vi "Write Nested Viewable Enqueuers.vi"(8 "error in (no error)":errorcluster, 9 "Viewable Names (optional)":string[](array[string]), 10 "Nested Viewable Enqueuers":refnum<class "Message Enqueuer.lvclass">[](array[class]), 11 "IViewManager In":refnum<class "IViewManager.lvclass">) -> (0 "error out":errorcluster, 3 "IViewManager Out":refnum<class "IViewManager.lvclass">)   [LabVIEW 2018, in "MVA Framework.lvlib" / "IViewManager.lvlib" / "IViewManager.lvclass"]
doc: "写入嵌套视图消息队列"
uses:
  IViewManager.lvclass
  <vilib>/ActorFramework/Message Enqueuer/Message Enqueuer.lvclass
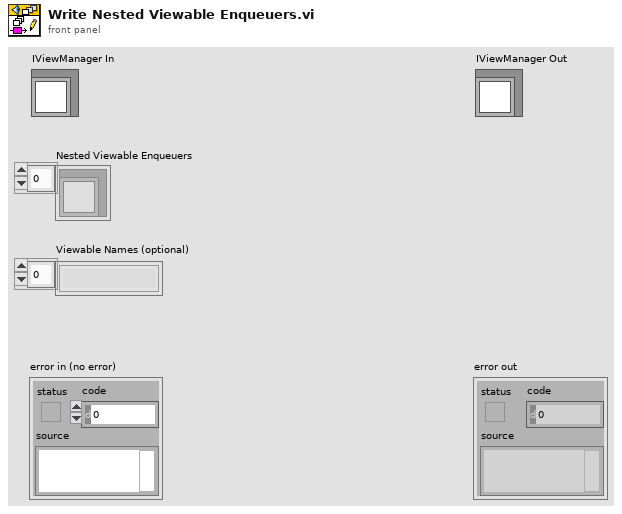
[diagram p1: front panel]
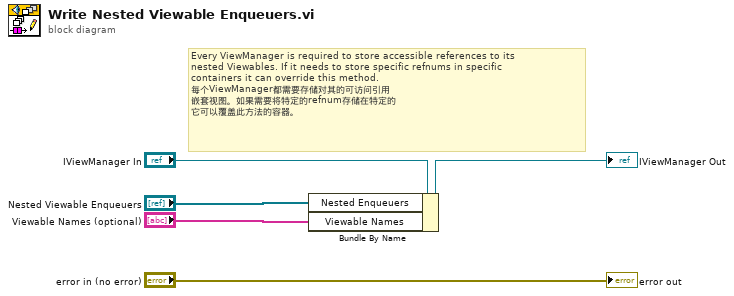
[diagram p0: block diagram]
diagram:
  # "Every ViewManager is required to store accessible references to its\nnested Viewables. If it needs to store specific refnums in specific\ncontainers it can override this method.\n每个ViewManager都需要存储对其的可访问引用\n嵌套视图。如果需要将特定的refnum存储在特定的\n它可以覆盖此方法的容器。"
  n1 = Bundle By Name(cluster="IViewManager In", "Nested Enqueuers"="Nested Viewable Enqueuers", "Viewable Names"="Viewable Names (optional)") -> (→"IViewManager Out":refnum<class "IViewManager.lvclass">)
  "error out" <- "error in (no error)"
